vi "DefaultFromINI.vi"(8 "error in (no error)":errorcluster, 11 "NhRegenGridSim":refnum<class "NHRGridSim.lvclass">) -> (0 "error out":errorcluster, 3 "NhRegenGridSim":refnum<class "NHRGridSim.lvclass">)   [LabVIEW 2018, in "AcPwrPlugins.lvlib" / "NHRGridSim.lvclass"]
doc: "This VI reads the properties from the INI file and puts them into the LabVIEW class for further use."
uses:
  NHRGridSim.lvclass
  C:/Program Files (x86)/National Instruments/LabVIEW 2018/user.lib/NIST/BaseClasses/BasePlugin_class/BasePlugin.lvclass
  C:/Users/Public/Projects/ICDAS/NistPluggableModules/AcPwr/AcPwrPlugins/AcPwrBaseClass/AcPwrBase.lvclass
  Measurements.ctl
  TypeDefs/MeasurementType.ctl
  TypeDefs/Device(s)Settings.ctl
  TypeDefs/Modules.ctl
  <userlib>/NIST/BaseClasses/BasePlugin_class/BasePlugin.lvclass/BasePlugin.ctl
  <userlib>/NIST/BaseClasses/BasePlugin_class/Accessors/Read PluginIniFilePath.vi
  AcPwrBaseClass/AcPwrBase.lvclass
  <vilib>/Utility/config.llb/NI_LVConfig.lvlib
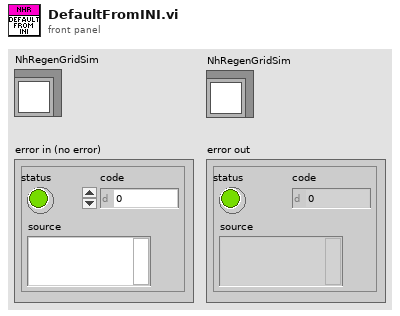
[diagram p1: front panel]
types:
  T1 = typedef "AcPwrPlugins.lvlib/NHRGridSim.lvclass/Device(s)Settings.ctl" = cluster{"MeasName":string, "Modules":T2}
  T2 = typedef "AcPwrPlugins.lvlib/NHRGridSim.lvclass/Modules.ctl" = cluster{"Measurement":cluster{"ApertureLength (s)":dbl, "NumberOfSamples":u32}, "Ranges":cluster{"Irange (A)":dbl, "Vrange (V)":dbl}, "Mode":u8, "Handle":string, "FreqOut (Hz)":dbl, "Connected":bool, "btnIdQuery":bool, "btnReset":bool, "Initialize Timeout ( ms)":u32, "Phase (0: All)":i32, "WatchDog":cluster{"Enable WatchDog":bool, "Robust WatchDog":bool, "Watchdog Interval (s)":dbl}, "Safety Limits":cluster{"Min Voltage (V)":dbl, "Min Voltage Time (s)":dbl, "Max Voltage (V)":dbl, "MaxVoltage Time (s)":dbl, "Max Source Amps (A)":dbl, "Max Source Amps Time (s)":dbl, "Max Sink Amps (A)":dbl, "Max Sink Amps Time (s)":dbl, "Max Source Power (W)":dbl, "Max Source Power Time (s)":dbl, "Max Sink Power (W)":dbl, "Max Sink Power Time (s)":dbl, "Peak Voltage (V)":dbl, "Peak Voltage Enable":bool, "Peak Amps (A)":dbl, "Peak Amps Enable":bool}, "Phases":cluster{"Pout (W)":dbl, "Iout (A)":dbl, "PhaseAngle":dbl, "Vout (V)":dbl, "Phase Name":string}[], "Regulation Gain":dbl, "ChangeOntheFly":bool, "Synchronize Output \nto Phase":bool, "Slew Rate":cluster{"Voltage Slew (Volts/s)":dbl, "Phase Angle (Degrees/s)":dbl}}[]
  T3 = typedef "AcPwrPlugins.lvlib/NHRGridSim.lvclass/Measurements.ctl" = cluster{"Handle":string, "Name":string, "Enabled ":bool, "Measurement Value":dbl, "Phase ":i32, "Measurement Type ":T4}[]
  T4 = typedef "AcPwrPlugins.lvlib/NHRGridSim.lvclass/MeasurementType.ctl" = enum16{"Average Current", "Average Voltage"}
  T5 = typedef "NI_LVConfig.lvlib/Config Data RefNum.ctl" = refnum<k1>
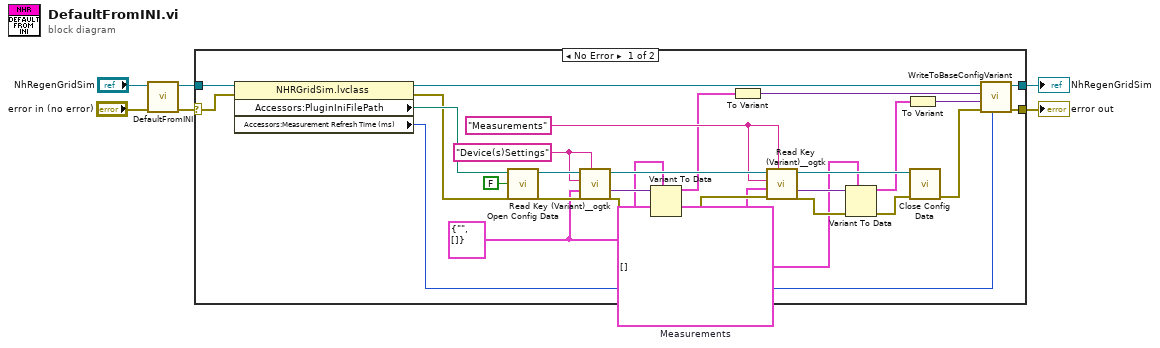
[diagram p0: block diagram]
diagram:
  n1 = call-parent "DefaultFromINI.vi"("error in (no error)"="error in (no error)", "AcPwrBase"="NhRegenGridSim") -> ("error out"=w1:errorcluster, "AcPwrBase"=w4:refnum<class "NHRGridSim.lvclass">)  [unwired: 8 in]
  n2 = case shown="No Error" w1 {
    selector: w1 -> [w26 w35]
    tunnel: w4 -> [w34 w36]
    tunnel: [w9 w36] -> w6
    tunnel: [w15 w35] -> w5
    frame No Error {
      w7 = T1 {"MeasName"="", "Modules"=[]} ("Device(s)Settings")
      w17 = T3 []  # Measurements
      w18 = "Measurements" ("section")
      w27 = "Device(s)Settings" ("section")
      n3 = property class="NHRGridSim.lvclass"(reference=w34, error in=w26) -> (reference out=w10:refnum<class "NHRGridSim.lvclass">, error out=w25:errorcluster, "Accessors:PluginIniFilePath"=w33:path, "Accessors:Measurement Refresh Time (ms)"=w8:u32)
      n4 = call <vilib>:"Open Config Data.vi"("error in (no error)"=w25, "create file if necessary (T)"=FALSE, "configuration file path"=w33) -> ("error out"=w30:errorcluster, "refnum"=w31:T5)  [unwired: 6 in, 1 out]
      n5 = call <userlib>:"Read Key (Variant)__ogtk.vi"("section"=w27, "error in (no error)"=w30, "type"=w7, "key (optional)"=w27, "refnum"=w31) -> ("error out"=w28:errorcluster, "key-value"=w29:variant, "refnum out"=w22:T5)  [unwired: 3 in, 1 out]
      n6 = Variant To Data(error in=w28, type=w7, Variant=w29) -> (data=w11:T1, error out=w19:errorcluster)
      n7 = To Variant(anything=w11) -> (Variant=w13:variant)
      n8 = call <userlib>:"Read Key (Variant)__ogtk.vi"("section"=w18, "error in (no error)"=w19, "type"=w17, "key (optional)"=w18, "refnum"=w22) -> ("error out"=w24:errorcluster, "key-value"=w23:variant, "refnum out"=w21:T5)  [unwired: 3 in, 1 out]
      n9 = Variant To Data(error in=w24, type=w17, Variant=w23) -> (data=w12:T3, error out=w20:errorcluster)
      n10 = To Variant(anything=w12) -> (Variant=w14:variant)
      n11 = call <vilib>:"Close Config Data.vi"("error in (no error)"=w20, "refnum"=w21) -> ("error out"=w16:errorcluster)  [unwired: 8 in, 1 out]
      n12 = call "WriteToBaseConfigVariant.vi"("Measurement RefreshTime (ms)"=w8, "error in (no error)"=w16, "Meas"=w14, "Config"=w13, "NHRGridSim in"=w10) -> ("error out"=w15:errorcluster, "NHRGridSim out"=w9:refnum<class "NHRGridSim.lvclass">)  [unwired: 5 in]
    }
    frame Error {
    }
  }
  "error out" <- w5
  "NhRegenGridSim" <- w6
